vi "Reset.vi"(8 "error in (no error)":errorcluster, 11 "AbstractCollector in":refnum<class "AbstractCollector.lvclass">) -> (0 "error out":errorcluster, 3 "AbstractCollector out":refnum<class "AbstractCollector.lvclass">)   [LabVIEW 2014, in "AbstractCollector.lvclass"]
uses:
  AbstractCollector.lvclass
  AbstractCollector.lvclass/AbstractCollector.ctl
  Interfaces/Observable Actor/Observable Actor.lvclass
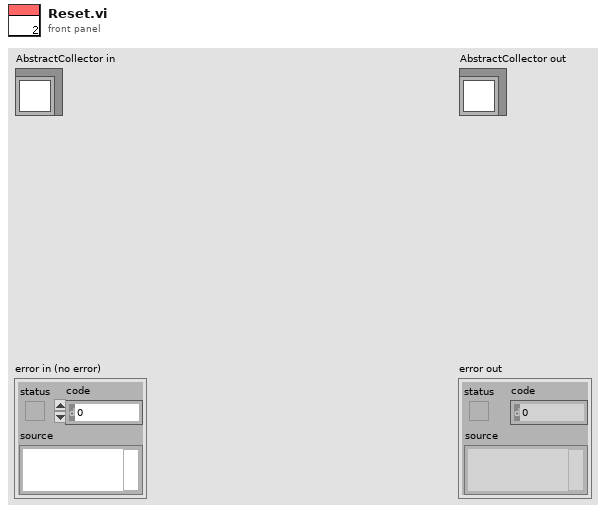
[diagram p1: front panel]
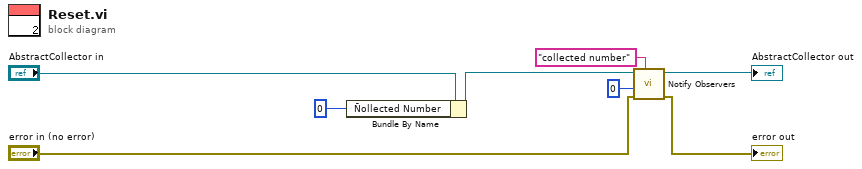
[diagram p0: block diagram]
diagram:
  n1 = Bundle By Name(cluster="AbstractCollector in", "Ñollected Number"=u32 0 ("#now")) -> (w6:refnum<class "AbstractCollector.lvclass">)
  n2 = call "Notify Observers.vi"("name"="collected number", "error in (no error)"="error in (no error)", "value"=u32 0 ("#now"), "Observable Actor in"=w6) -> ("error out"=→"error out":errorcluster, "Observable Actor out"=→"AbstractCollector out":refnum<class "AbstractCollector.lvclass">)  [unwired: 6 in]
